vi "CRYComplex Binary Operation.vi"(4 "Axis Mode":u16(slide), 6 "A data for units":T1={"Name"="", "Curve"=[], "X data"=1, "Y data"=1, "Z data"=1, "X axis"=0, "Y axis"=1, "Z axis"=1, "X unit"="Hz", "Y unit"="", "Z unit"="deg.", "X dB ref"=1.0, "Y dB ref"=1.0, "Z dB ref"=1.0, "single val"=FALSE, "protected"=FALSE, "display X"=TRUE, "display Y"=TRUE, "display Z"=TRUE, "Test Info"="", "Step No."=0, "Plot Settings"={"Color"=0, "Interpolation"=0, "Point Style"=0, "Line Style"=0, "Point Color"=0, "Line Width"=0, "Bar Plot Style"=0, "Fill To"=0}, "AutoProtect"=FALSE} {"Z data" items=["dB", "Lin"]; "X data" items=["dB", "Lin"]; "Y data" items=["dB", "Lin"]; "Z dB ref" format="%.1f"; "Z axis" items=["Log", "Lin"]; "X dB ref" format="%.1f"; "X axis" items=["Log", "Lin"]; "Y axis" items=["Log", "Lin"]; "Y dB ref" format="%.1f"; "Curve"."z" format="%.2f"; "Curve"."y" format="%.2f"; "Curve"."x" format="%.2f"}, 7 "B data for units":T1={"Name"="", "Curve"=[], "X data"=1, "Y data"=1, "Z data"=1, "X axis"=0, "Y axis"=1, "Z axis"=1, "X unit"="Hz", "Y unit"="", "Z unit"="deg.", "X dB ref"=1.0, "Y dB ref"=1.0, "Z dB ref"=1.0, "single val"=FALSE, "protected"=FALSE, "display X"=TRUE, "display Y"=TRUE, "display Z"=TRUE, "Test Info"="", "Step No."=0, "Plot Settings"={"Color"=0, "Interpolation"=0, "Point Style"=0, "Line Style"=0, "Point Color"=0, "Line Width"=0, "Bar Plot Style"=0, "Fill To"=0}, "AutoProtect"=FALSE} {"Z data" items=["dB", "Lin"]; "X data" items=["dB", "Lin"]; "Y data" items=["dB", "Lin"]; "Z dB ref" format="%.1f"; "Z axis" items=["Log", "Lin"]; "X dB ref" format="%.1f"; "X axis" items=["Log", "Lin"]; "Y axis" items=["Log", "Lin"]; "Y dB ref" format="%.1f"; "Curve"."z" format="%.2f"; "Curve"."y" format="%.2f"; "Curve"."x" format="%.2f"}, 8 "Curve B":cluster{"x":dbl, "y":dbl, "z":dbl}[](array[cluster]) {"z" format="%.2f"; "y" format="%.2f"; "x" format="%.2f"}, 9 "operator":u16(ring) items=["+", "--", "x", "/"], 10 "Work in":u16(slide), 11 "Curve A":cluster{"x":dbl, "y":dbl, "z":dbl}[](array[cluster]) {"z" format="%.2f"; "y" format="%.2f"; "x" format="%.2f"}) -> (0 "Single val out":bool, 1 "Result dB ref":dbl=1.0 format="%.1f", 2 "Result Y unit":string, 3 "Result":cluster{"x":dbl, "y":dbl, "z":dbl}[](array[cluster]) {"z" format="%.2f"; "y" format="%.2f"; "x" format="%.2f"})   [LabVIEW 2013]
uses:
  Typedef Control/CRYData Cluster.ctl
panel:
  # "="
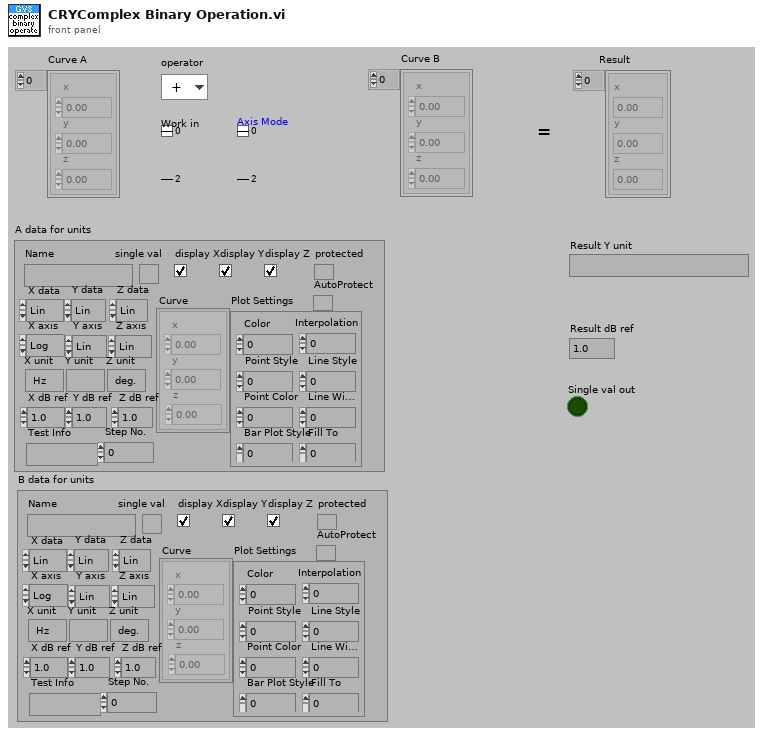
[diagram p1: front panel]
types:
  T1 = typedef "CRYData Cluster.ctl" = cluster{"Name":string, "Curve":cluster{"x":dbl, "y":dbl, "z":dbl}[], "X data":u16, "Y data":u16, "Z data":u16, "X axis":u16, "Y axis":u16, "Z axis":u16, "X unit":string, "Y unit":string, "Z unit":string, "X dB ref":dbl, "Y dB ref":dbl, "Z dB ref":dbl, "single val":bool, "protected":bool, "display X":bool, "display Y":bool, "display Z":bool, "Test Info":string, "Step No.":i32, "Plot Settings":cluster{"Color":u32, "Interpolation":u8, "Point Style":u8, "Line Style":u8, "Point Color":u32, "Line Width":u8, "Bar Plot Style":u8, "Fill To":i16}, "AutoProtect":bool}
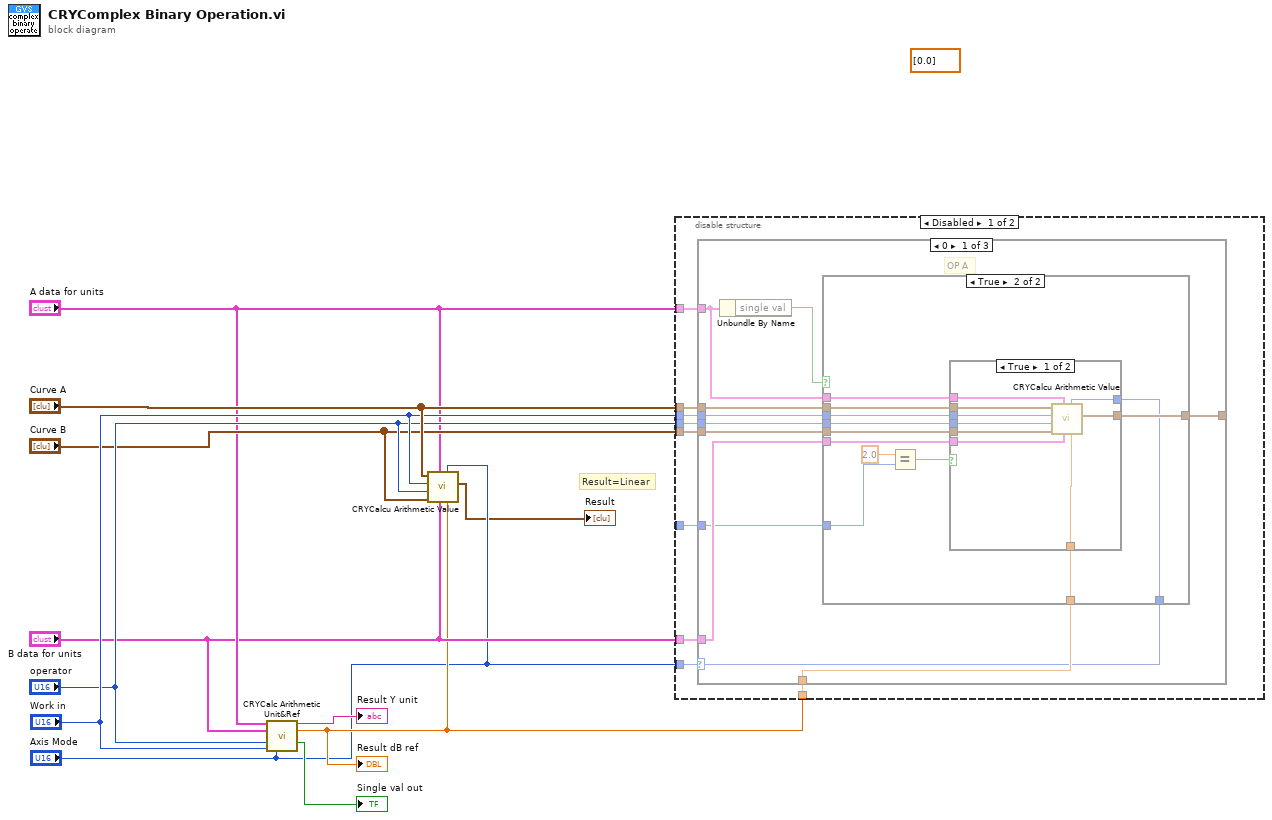
[diagram p0: block diagram]
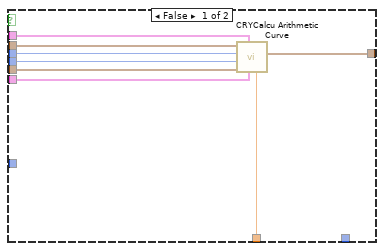
[diagram p2: hidden frame]
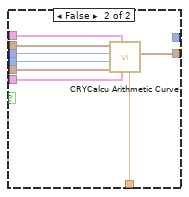
[diagram p3: hidden frame]
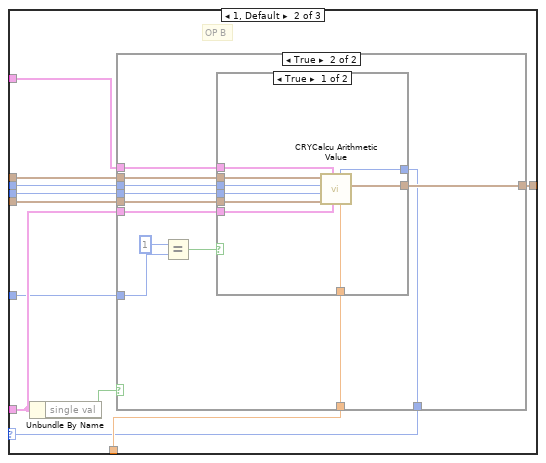
[diagram p4: hidden frame]
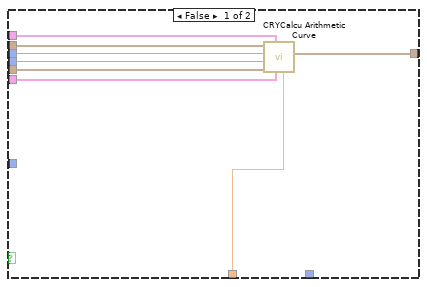
[diagram p5: hidden frame]
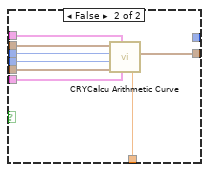
[diagram p6: hidden frame]
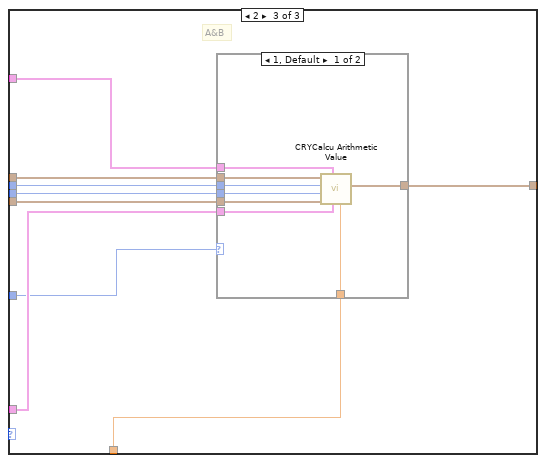
[diagram p7: hidden frame]
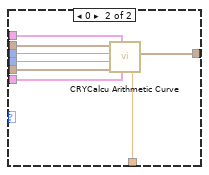
[diagram p8: hidden frame]
diagram:
  (unwired) dbl[] [0.0]
  # "Result=Linear"
  n1 = call "CRYCalc Arithmetic Unit&Ref.vi"("A data for units"="A data for units", "B data for units"="B data for units", "operator"="operator", "Work in"="Work in", "Axis Mode"="Axis Mode") -> ("Result Y unit"=→"Result Y unit":string, "Result dB ref(A)"=w3:dbl, "Single val out"=→"Single val out":bool)  [unwired: 5 in, 3 out]
  "Result dB ref" <- w3
  n2 = call "CRYCalcu Arithmetic Value.vi"("dB ref"=w3, "Axis Mode"="Axis Mode", "B data for units"="B data for units", "A data for units"="A data for units", "Curve B"="Curve B", "operator"="operator", "Work in"="Work in", "Curve A"="Curve A") -> ("Result"=→"Result":cluster{"x":dbl, "y":dbl, "z":dbl}[])  [unwired: 3 in]
  n3 = disable-structure shown="Disabled" {
    disable-tunnel: "Curve A" -> [w20 _]
    disable-tunnel: "Curve B" -> [w19 _]
    disable-tunnel: "Work in" -> [w18 _]
    disable-tunnel: "operator" -> [w17 _]
    disable-tunnel: w3 -> [w16 _]
    disable-tunnel: "Axis Mode" -> [w15 _]
    disable-tunnel: "A data for units" -> [w14 _]
    disable-tunnel: "B data for units" -> [w13 _]
    disable-tunnel: _ -> [w12 _]
    frame Disabled {
      n4 = case shown="0" w15 {
        selector: w15 -> [w22 w70 _]
        tunnel: w20 -> [w30 w77 w124]
        tunnel: w19 -> [w29 w74 w121]
        tunnel: w18 -> [w27 w76 w123]
        tunnel: w17 -> [w28 w75 w122]
        tunnel: w14 -> [w26 w78 w125]
        tunnel: w13 -> [w25 w73 w120]
        tunnel: w16 -> [w24 w72 w119]
        tunnel: [w23 w71 w118] -> _
        tunnel: w12 -> [w21 w69 w117]
        frame 0 {
          # "OP A"
          n5 = Unbundle By Name(w26) -> ("single val"=w31:bool)
          n6 = case shown="True" w31 {
            tunnel: w30 -> [w39 w51]
            tunnel: w29 -> [w38 w40]
            tunnel: w28 -> [w37 w50]
            tunnel: w27 -> [w36 w49]
            tunnel: w26 -> [w35 w48]
            tunnel: w25 -> [w34 w47]
            tunnel: w24 -> [w33 w46]
            tunnel: [w32 w45] -> w23
            tunnel: w22 -> [_ w44]
            tunnel: w21 -> [_ w42]
            frame False {
              n7 = call "CRYCalcu Arithmetic Curve.vi"("dB ref"=w33, "B data for units"=w34, "A data for units"=w35, "Curve B"=w38, "operator"=w37, "Work in"=w36, "Curve A"=w39) -> ("Result"=w32:cluster{"x":dbl, "y":dbl, "z":dbl}[])  [unwired: 4 in]
            }
            frame True {
              n8 = Equal?(x=2.0, y=w42) -> (x = y?=w41:bool)
              n9 = case shown="True" w41 {
                tunnel: w51 -> [w60 w68]
                tunnel: w50 -> [w59 w67]
                tunnel: w49 -> [w58 w66]
                tunnel: w48 -> [w57 w65]
                tunnel: w47 -> [w56 w64]
                tunnel: w46 -> [w55 w63]
                tunnel: [w54 w62] -> w45
                tunnel: w44 -> [w53 _]
                tunnel: w40 -> [w52 w61]
                frame True {
                  n10 = call "CRYCalcu Arithmetic Value.vi"("dB ref"=w55, "Axis Mode"=w53, "B data for units"=w56, "A data for units"=w57, "Curve B"=w52, "operator"=w59, "Work in"=w58, "Curve A"=w60) -> ("Result"=w54:cluster{"x":dbl, "y":dbl, "z":dbl}[])  [unwired: 3 in]
                }
                frame False {
                  n11 = call "CRYCalcu Arithmetic Curve.vi"("dB ref"=w63, "B data for units"=w64, "A data for units"=w65, "Curve B"=w61, "operator"=w67, "Work in"=w66, "Curve A"=w68) -> ("Result"=w62:cluster{"x":dbl, "y":dbl, "z":dbl}[])  [unwired: 4 in]
                }
              }
            }
          }
        }
        frame 1, Default {
          # "OP B"
          n12 = Unbundle By Name(w73) -> ("single val"=w79:bool)
          n13 = case shown="True" w79 {
            tunnel: w77 -> [w80 w99]
            tunnel: w74 -> [w87 w98]
            tunnel: w75 -> [w86 w97]
            tunnel: w76 -> [w85 w96]
            tunnel: w78 -> [w84 w95]
            tunnel: w73 -> [w83 w94]
            tunnel: w72 -> [w82 w93]
            tunnel: [w81 w92] -> w71
            tunnel: w70 -> [_ w91]
            tunnel: w69 -> [_ w88]
            frame False {
              n14 = call "CRYCalcu Arithmetic Curve.vi"("dB ref"=w82, "B data for units"=w83, "A data for units"=w84, "Curve B"=w87, "operator"=w86, "Work in"=w85, "Curve A"=w80) -> ("Result"=w81:cluster{"x":dbl, "y":dbl, "z":dbl}[])  [unwired: 4 in]
            }
            frame True {
              n15 = Equal?(x=i8 1, y=w88) -> (x = y?=w90:bool)
              n16 = case shown="True" w90 {
                tunnel: w99 -> [w100 w116]
                tunnel: w98 -> [w101 w115]
                tunnel: w97 -> [w108 w114]
                tunnel: w96 -> [w107 w113]
                tunnel: w95 -> [w106 w112]
                tunnel: w94 -> [w105 w111]
                tunnel: w93 -> [w104 w110]
                tunnel: [w103 w109] -> w92
                tunnel: w91 -> [w102 _]
                frame True {
                  n17 = call "CRYCalcu Arithmetic Value.vi"("dB ref"=w104, "Axis Mode"=w102, "B data for units"=w105, "A data for units"=w106, "Curve B"=w101, "operator"=w108, "Work in"=w107, "Curve A"=w100) -> ("Result"=w103:cluster{"x":dbl, "y":dbl, "z":dbl}[])  [unwired: 3 in]
                }
                frame False {
                  n18 = call "CRYCalcu Arithmetic Curve.vi"("dB ref"=w110, "B data for units"=w111, "A data for units"=w112, "Curve B"=w115, "operator"=w114, "Work in"=w113, "Curve A"=w116) -> ("Result"=w109:cluster{"x":dbl, "y":dbl, "z":dbl}[])  [unwired: 4 in]
                }
              }
            }
          }
        }
        frame 2 {
          # "A&B"
          n19 = case shown="1, Default" w117 {
            tunnel: w124 -> [w126 w141]
            tunnel: w121 -> [w127 w140]
            tunnel: w122 -> [w133 w139]
            tunnel: w123 -> [w132 w138]
            tunnel: w125 -> [w131 w137]
            tunnel: w120 -> [w130 w136]
            tunnel: w119 -> [w129 w135]
            tunnel: [w128 w134] -> w118
            frame 1, Default {
              n20 = call "CRYCalcu Arithmetic Value.vi"("dB ref"=w129, "B data for units"=w130, "A data for units"=w131, "Curve B"=w127, "operator"=w133, "Work in"=w132, "Curve A"=w126) -> ("Result"=w128:cluster{"x":dbl, "y":dbl, "z":dbl}[])  [unwired: 4 in]
            }
            frame 0 {
              n21 = call "CRYCalcu Arithmetic Curve.vi"("dB ref"=w135, "B data for units"=w136, "A data for units"=w137, "Curve B"=w140, "operator"=w139, "Work in"=w138, "Curve A"=w141) -> ("Result"=w134:cluster{"x":dbl, "y":dbl, "z":dbl}[])  [unwired: 4 in]
            }
          }
        }
      }
    }
    frame Enabled {
    }
  }
